vi "5790A_guard.vi"(2 "error in":errorcluster, 3 "Guard Connection (T: external)":bool, 5 "5790A":refnum<visa-resource-name>) -> (0 "error out":errorcluster, 1 "Session Out":refnum<visa-resource-name>)   [LabVIEW 2020]
uses:
  <vilib>/Instr/_visa.llb/VISA GPIB Control REN Mode.ctl
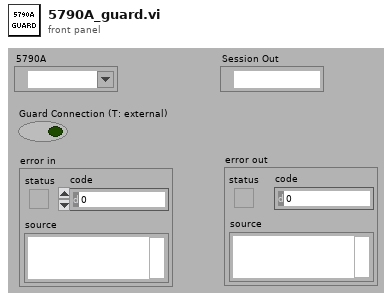
[diagram p1: front panel]
types:
  T1 = typedef "VISA GPIB Control REN Mode.ctl" = u16
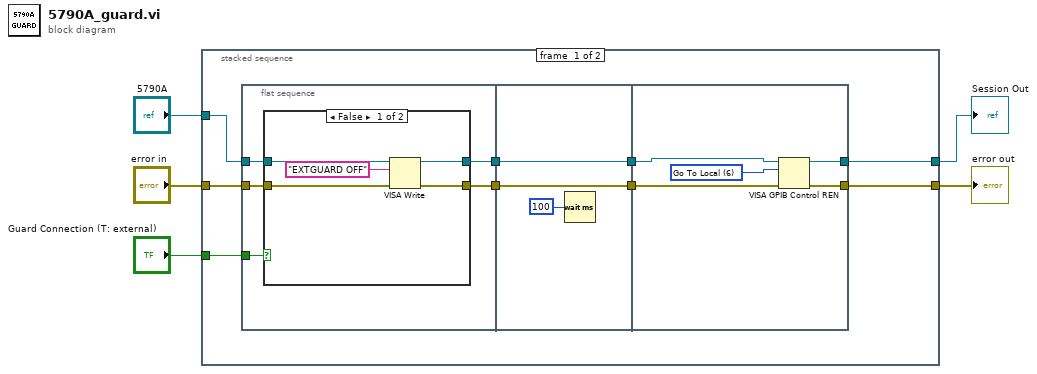
[diagram p0: block diagram]
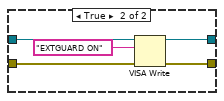
[diagram p2: hidden frame]
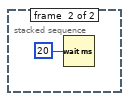
[diagram p3: hidden frame]
diagram:
  n1 = stacked-sequence {
    tunnel: "5790A" -> [w14 _]
    tunnel: "Guard Connection (T: external)" -> [w13 _]
    tunnel: "error in" -> [w12 _]
    tunnel: [w11 _] -> w4
    tunnel: [w10 _] -> w5
    frame #0 {
      n2 = flat-sequence {
        tunnel: w13 -> [w19]
        tunnel: [w17] -> w9
        tunnel: [w18] -> w7
        tunnel: w14 -> [w16]
        tunnel: w12 -> [w15]
        tunnel: w9 -> [w32]
        tunnel: [w32] -> w8
        tunnel: w7 -> [w31]
        tunnel: [w31] -> w6
        tunnel: [w34] -> w10
        tunnel: [w33] -> w11
        tunnel: w8 -> [w36]
        tunnel: w6 -> [w35]
        frame #0 {
          n3 = case shown="False" w19 {
            tunnel: [w23 w29] -> w18
            tunnel: [w22 w28] -> w17
            tunnel: w16 -> [w24 w27]
            tunnel: w15 -> [w21 w26]
            frame False {
              n4 = VISA Write(VISA resource name=w24, write buffer="EXTGUARD OFF", error in (no error)=w21) -> (VISA resource name out=w23:refnum<visa-resource-name>, error out=w22:errorcluster)  [unwired: 1 out]
            }
            frame True {
              n5 = VISA Write(VISA resource name=w27, write buffer="EXTGUARD ON", error in (no error)=w26) -> (VISA resource name out=w29:refnum<visa-resource-name>, error out=w28:errorcluster)  [unwired: 1 out]
            }
          }
        }
        frame #1 {
          n6 = Wait (ms)(milliseconds to wait=u32 100 ("millisecond multiple")) -> ()  [unwired: 1 out]
        }
        frame #2 {
          w37 = T1 6 items=["Deassert REN", "Assert REN", "Go To Local; Deassert REN ", "Assert REN; Address Device", "Local Lockout (Addressed Devices)", "Local Lockout (This Device)", "Go To Local"] ("Mode")
          n7 = VISA GPIB Control REN(8:w36, 10:w37, 11:w35) -> (0:w33:errorcluster, 3:w34:refnum<visa-resource-name>)
        }
      }
    }
    frame #1 {
      n8 = Wait (ms)(milliseconds to wait=u32 20 ("millisecond multiple")) -> ()  [unwired: 1 out]
    }
  }
  "Session Out" <- w5
  "error out" <- w4
